vi "XW_Map_Global.vi"() -> ()   [LabVIEW 2010]
uses:
  Map method.ctl
panel:
  out "All nodes processed and processed without error":bool
  in  "Pad":dbl=1.01
  in  "Apply calibration corrections":bool=TRUE
  out "pts per set":i32
  in  "Map method":T1=enum."Const. Psi_eff (std.)"
  in  "cap indicial sum to n":bool=TRUE
  out "no. of pts outside map":i32
  in  "Coerced surface order":i32
  # "Trimesh mode only:"
  # "Polynomial surface method only:"
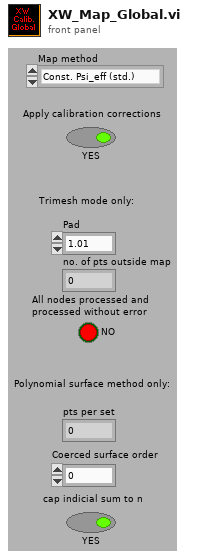
[diagram p1: front panel]
types:
  T1 = typedef "Map method.ctl" = enum16{"Triangle mesh", "Polynomial surface", "Const. Psi_eff (std.)", "Psi_eff = f(Umagn.)", "Psi_eff, k = f(Umagn.)"}
diagram:
